vi "Main.vi"() -> ()   [LabVIEW 2020]
doc: "Use this template to build a simple state machine design pattern. Each state executes code and determines which state to transition to."
uses:
  controls/ICM-LOG State.ctl
  controls/ICM-LOG Data.ctl
panel:
  out "Top Label":string
  in  "Tab Control":T1(tab)
  in  "Export definition":bool
  in  "delete definition":bool
  in  "Import definition":bool
  in  "Definition Type":u16(ring) items=["Choose a Definition", "device", "module", "channel", "metric", "instance", "unit", "asset", "datasource", "capability", "camera"]
  in  "Definition List":i32(listbox)
  in  "Export Asset":bool
  in  "Import Asset":bool
  in  "Asset Configuration File Path":path
  in  "Asset":string="Equipment"
  in  "Start Date/Time":timestamp=timestamp(3664461539.734 s since 1904-01-01)
  in  "End Date/Time":timestamp=timestamp(3664465840.411149 s since 1904-01-01)
  in  "Destination Folder":path=path "C:/TDMS_Logs"
  in  "File List":i32(listbox)=-1
  in  "Pull Data":bool
  in  "Exit":bool
  out "Status":string="Exported 0 files to C:\\TDMS_Logs."
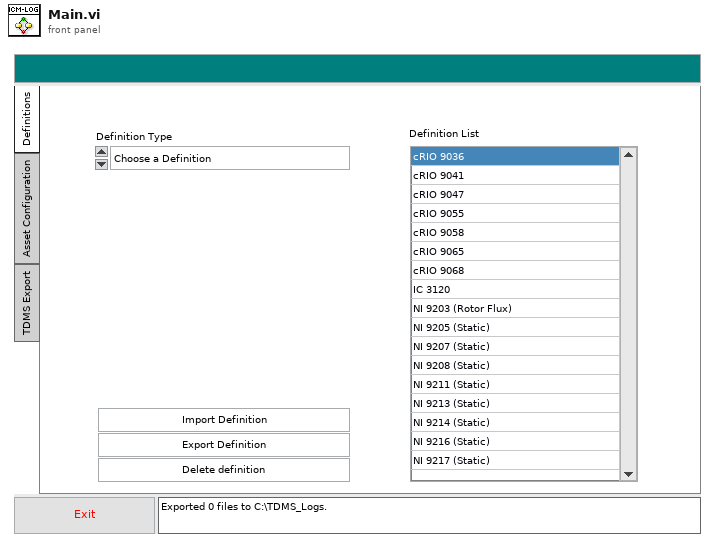
[diagram p1: front panel]
types:
  T1 = enum32{"Definitions", "Asset Configuration", "TDMS Export"}
  T2 = typedef "ICM-LOG Data.ctl" = cluster{"Asset":string, "Start Date/Time":timestamp, "End Date/Time":timestamp, "Destination Folder":path, "Command":string, "Standard Output":string, "filename":string, "Item Name":string, "GUID":string}
  T3 = typedef "ICM-LOG State.ctl" = enum16{"Initialize", "Wait for Event", "List Definitions", "Import Definition", "Export Definition", "Delete Definition", "Export Asset Configuration", "Import Asset Configuration", "Build Command", "Run Command", "Update Definition List", "Update File List", "Open File", "Exit"}
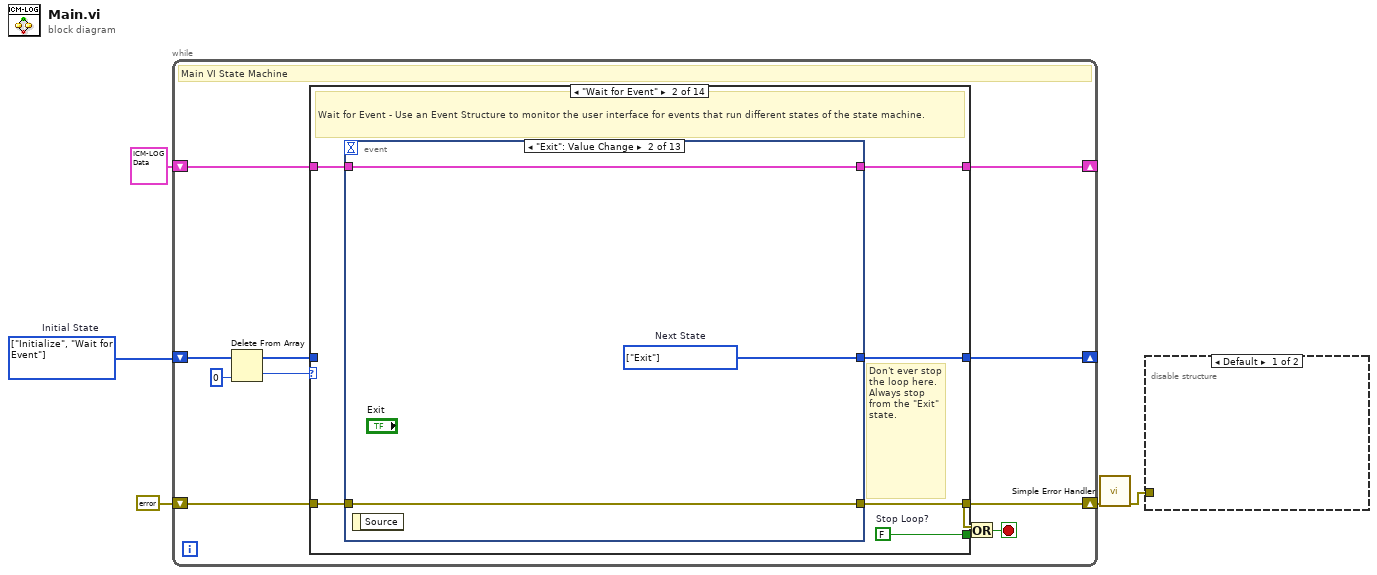
[diagram p0: block diagram]
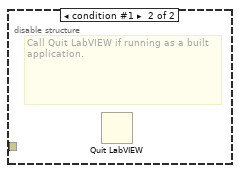
[diagram p2: hidden frame]
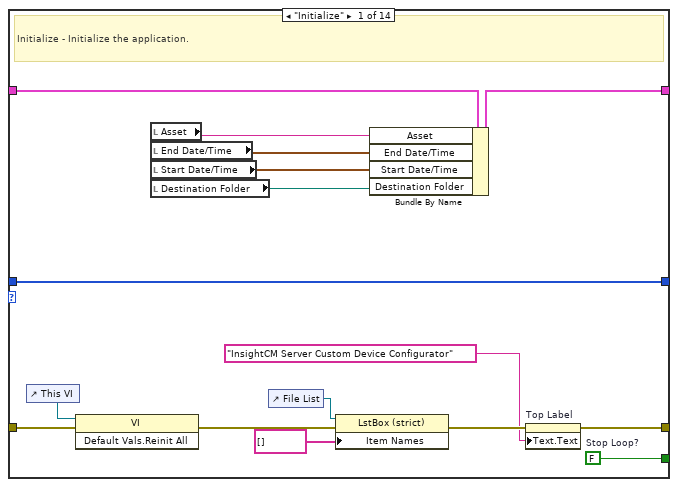
[diagram p3: hidden frame]
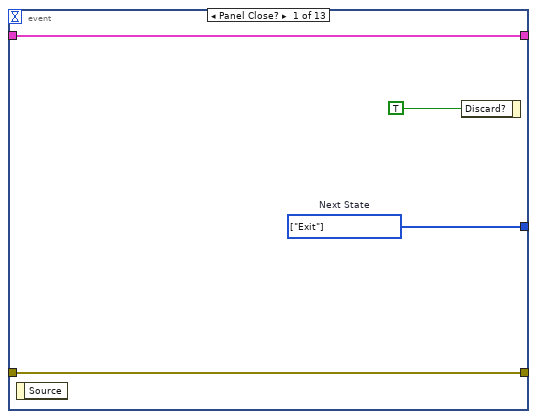
[diagram p4: hidden frame]
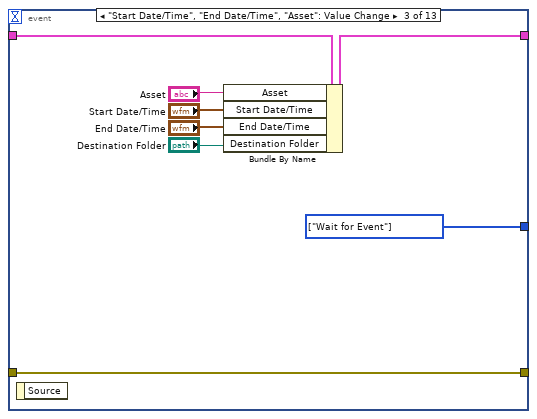
[diagram p5: hidden frame]
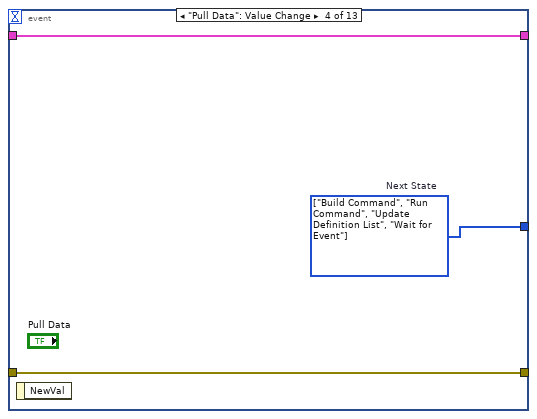
[diagram p6: hidden frame]
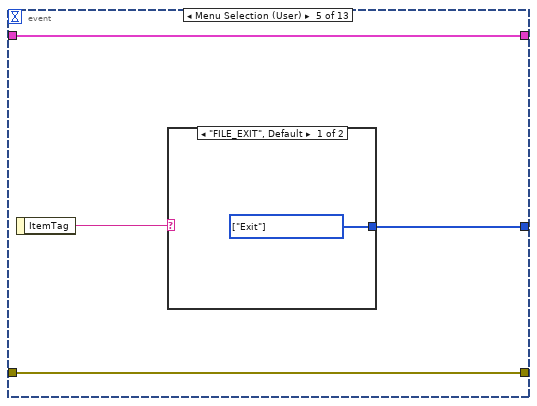
[diagram p7: hidden frame]
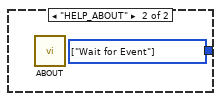
[diagram p8: hidden frame]
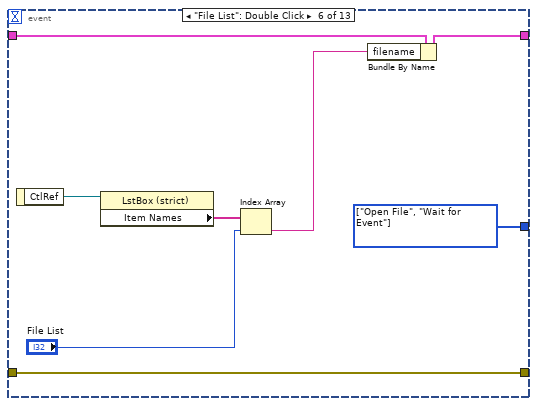
[diagram p9: hidden frame]
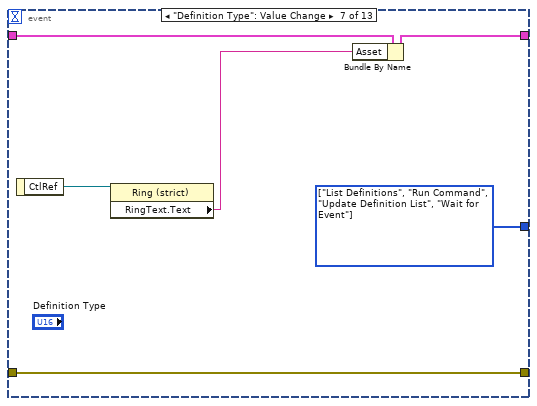
[diagram p10: hidden frame]
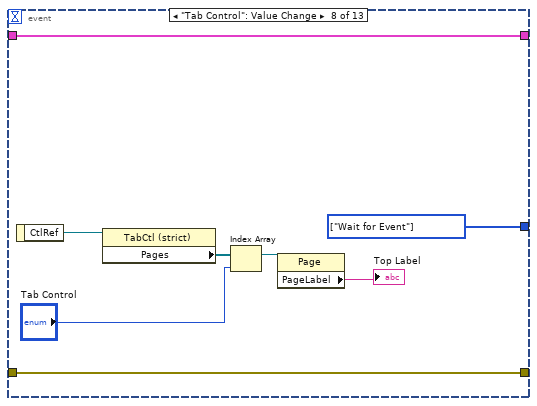
[diagram p11: hidden frame]
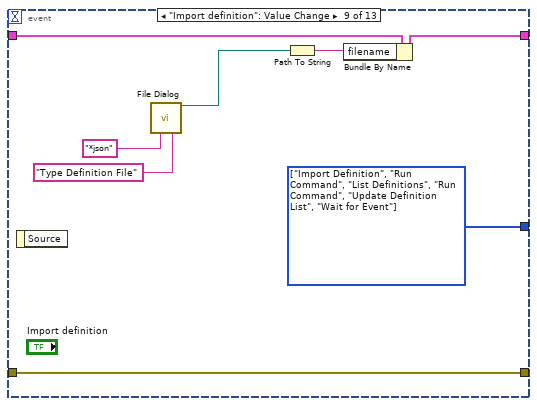
[diagram p12: hidden frame]
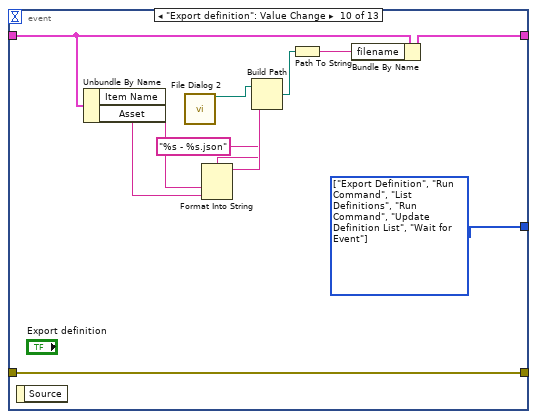
[diagram p13: hidden frame]
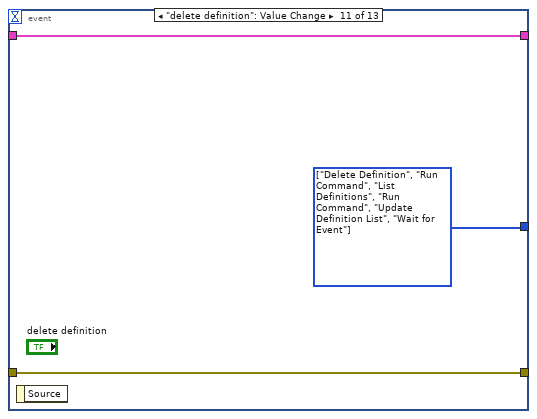
[diagram p14: hidden frame]
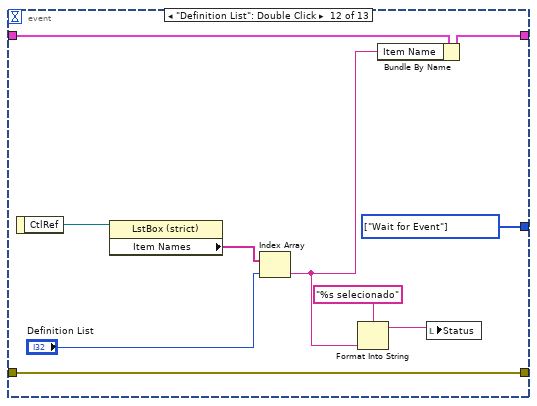
[diagram p15: hidden frame]
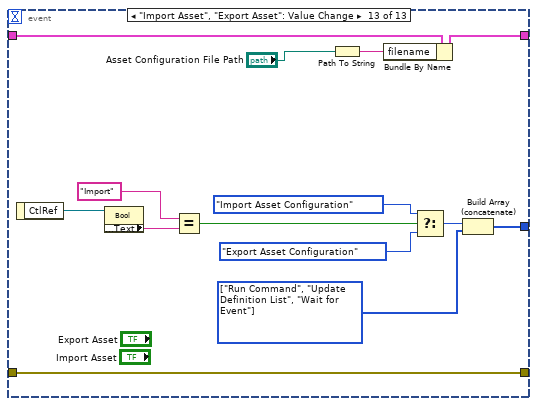
[diagram p16: hidden frame]
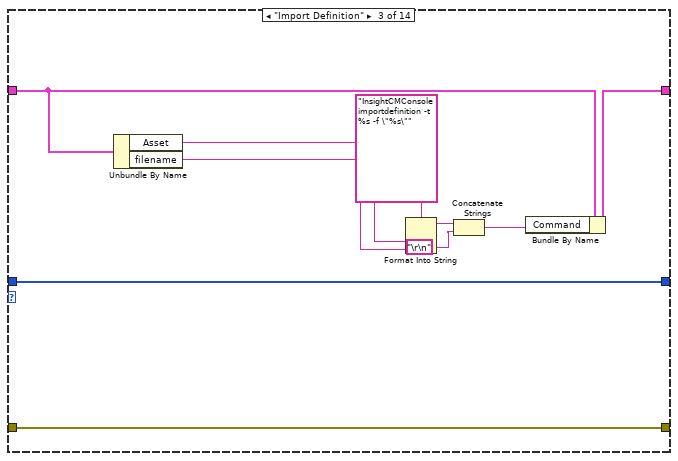
[diagram p17: hidden frame]
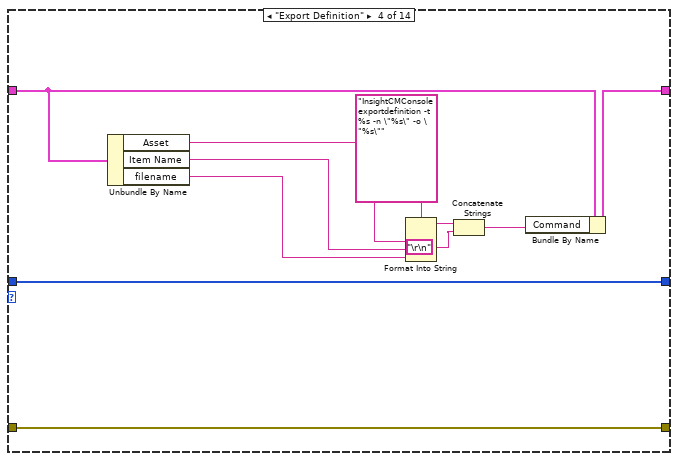
[diagram p18: hidden frame]
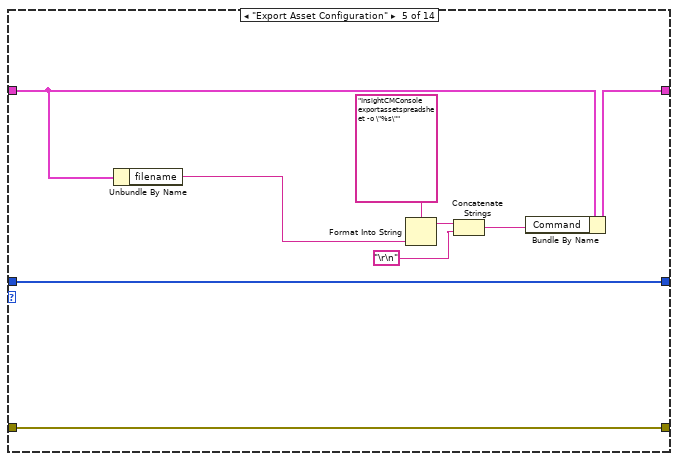
[diagram p19: hidden frame]
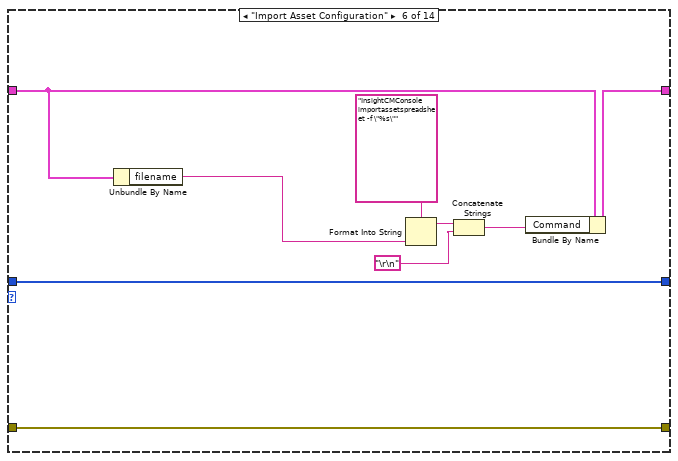
[diagram p20: hidden frame]
diagram:
  w5 = T3[] [enum."Initialize", enum."Wait for Event"] items=["Initialize", "Wait for Event", "List Definitions", "Import Definition", "Export Definition", "Delete Definition", "Export Asset Configuration", "Import Asset Configuration", "Build Command", "Run Command", "Update Definition List", "Update File List", "Open File", "Exit"]  # Initial State
  n1 = while {
    shift-right: [w7] -> _
    shift-left: w5 -> [w10]
    shift-right: [w15] -> _
    shift-left: T2 {"Asset"="", "Start Date/Time"=timestamp(0 s since 1904-01-01), "End Date/Time"=timestamp(0 s since 1904-01-01), "Destination Folder"=path "C:/TDMS_Logs", "Command"="", "Standard Output"="", "filename"="", "Item Name"="", "GUID"=""} ("Data") -> [w16]
    shift-right: [w11] -> w2
    shift-left: errorcluster {"status"=FALSE, "code"=0, "source"=""} ("error constant") -> [w14]
    stop <- w12 stop-if-true
    # "Main VI State Machine"
    n2 = Delete From Array(array=w10, index=0) -> (deleted portion=w9:T3, array with subset deleted=w8:T3[])  [unwired: 1 in]
    n3 = case shown="\"Wait for Event\"" w9 {
      tunnel: [w17 w38 w131 w141 w152 w161 w170 w180 w189 w206 w218 w240 w248 w258] -> w7
      tunnel: [w20 w37 _ _ _ _ _ _ _ FALSE ("Stop Loop?") _ _ _ w256] -> w13
      tunnel: w16 -> [w32 w36 w139 w150 w159 w168 w178 w187 w204 w216 w233 w246 w253 w257]
      tunnel: [w30 w35 w135 w147 w157 w166 w175 w185 w193 w209 w233 w246 w253 w257] -> w15
      tunnel: w14 -> [w31 w34 w140 w151 w160 w169 w179 w188 w205 w213 w234 w247 w254 w255]
      tunnel: [w19 w33 w140 w151 w160 w169 w179 w188 w205 w212 w234 w247 w250 w255] -> w11
      tunnel: w8 -> [w17 _ w131 w141 w152 w161 w170 w180 w189 w206 w218 w240 w248 _]
      frame "Initialize" {
        w20 = FALSE  # Stop Loop?
        # "Initialize - Initialize the application."
        n4 = control-ref of="This VI"() -> (w24:refnum<vi>)
        n5 = invoke class="VI" method="Default Vals.Reinit All"(reference=w24, error in=w31) -> (error out=w25:errorcluster)  [unwired: 1 in, 2 out]
        n6 = local read "Asset"() -> (w29:string)
        n7 = local read "End Date/Time"() -> (w28:timestamp)
        n8 = local read "Start Date/Time"() -> (w27:timestamp)
        n9 = local read "Destination Folder"() -> (w26:path)
        n10 = control-ref of="File List"() -> (w22:refnum<vi>)
        n11 = property class="LstBox (strict)"(reference=w22, error in=w25, "Item Names"=string[] []) -> (error out=w23:errorcluster)  [unwired: 1 out]
        n12 = Bundle By Name(cluster=w32, "Asset"=w29, "End Date/Time"=w28, "Start Date/Time"=w27, "Destination Folder"=w26) -> (w30:T2)
        n13 = property on="Top Label" class="Str"(error in=w23, "Text.Text"="InsightCM Server Custom Device Configurator" ("Top Label")) -> (error out=w19:errorcluster)  [unwired: 1 in, 1 out]
      }
      frame "Wait for Event" {
        w37 = FALSE  # Stop Loop?
        # "Don't ever stop the loop here. Always stop from the \"Exit\" state."
        # "Wait for Event - Use an Event Structure to monitor the user interface for events that run different states of the state machine."
        n14 = event shown="[1] \"Exit\": Value Change" {
          selector: _ -> [_ _ _ _ _ _ _ _ _ _ _ _ _]
          dyn-events: _ -> [_ _ _ _ _ _ _ _ _ _ _ _ _]
          timeout: _ -> [_ _ _ _ _ _ _ _ _ _ _ _ _]
          tunnel: [w42 w45 w46 w56 w57 w68 w74 w77 w89 w93 w104 w107 w117] -> w38
          tunnel: w36 -> [w41 w44 w53 w55 w60 w70 w76 w84 w88 w94 w106 w116 w130]
          tunnel: [w41 w44 w51 w55 w60 w64 w72 w84 w91 w102 w106 w111 w128] -> w35
          tunnel: w34 -> [w40 w43 w52 w54 w59 w69 w75 w83 w92 w103 w105 w115 w129]
          tunnel: [w40 w43 w52 w54 w59 w69 w75 w83 w92 w103 w105 w115 w129] -> w33
          event Panel Close? {
            w42 = T3[] [enum."Exit"] items=["Initialize", "Wait for Event", "List Definitions", "Import Definition", "Export Definition", "Delete Definition", "Export Asset Configuration", "Import Asset Configuration", "Build Command", "Run Command", "Update Definition List", "Update File List", "Open File", "Exit"]  # Next State
            n15 = event-data() -> ()  [unwired: 1 in, 1 out]
            n16 = event-data("Discard?"=TRUE) -> ()  [unwired: 1 in, 1 out]
          }
          event "Exit": Value Change {
            w45 = T3[] [enum."Exit"] items=["Initialize", "Wait for Event", "List Definitions", "Import Definition", "Export Definition", "Delete Definition", "Export Asset Configuration", "Import Asset Configuration", "Build Command", "Run Command", "Update Definition List", "Update File List", "Open File", "Exit"]  # Next State
            n17 = event-data() -> ()  [unwired: 1 in, 1 out]
          }
          event "Start Date/Time", "End Date/Time", "Asset": Value Change {
            w46 = T3[] [enum."Wait for Event"] items=["Initialize", "Wait for Event", "List Definitions", "Import Definition", "Export Definition", "Delete Definition", "Export Asset Configuration", "Import Asset Configuration", "Build Command", "Run Command", "Update Definition List", "Update File List", "Open File", "Exit"] ("Next State")
            n18 = event-data() -> ()  [unwired: 1 in, 1 out]
            n19 = Bundle By Name(cluster=w53, "Asset"="Asset", "Start Date/Time"="Start Date/Time", "End Date/Time"="End Date/Time", "Destination Folder"="Destination Folder") -> (w51:T2)
          }
          event "Pull Data": Value Change {
            w56 = T3[] [enum."Build Command", enum."Run Command", enum."Update Definition List", enum."Wait for Event"] items=["Initialize", "Wait for Event", "List Definitions", "Import Definition", "Export Definition", "Delete Definition", "Export Asset Configuration", "Import Asset Configuration", "Build Command", "Run Command", "Update Definition List", "Update File List", "Open File", "Exit"]  # Next State
            n20 = event-data() -> ()  [unwired: 1 in, 1 out]
          }
          event Menu Selection (User) {
            n21 = event-data() -> ("ItemTag"=w58:string)  [unwired: 1 in]
            n22 = case shown="\"FILE_EXIT\", Default" w58 {
              tunnel: [w61 w62] -> w57
              frame "FILE_EXIT", Default {
                w61 = T3[] [enum."Exit"] items=["Initialize", "Wait for Event", "List Definitions", "Import Definition", "Export Definition", "Delete Definition", "Export Asset Configuration", "Import Asset Configuration", "Build Command", "Run Command", "Update Definition List", "Update File List", "Open File", "Exit"] ("Next State")
              }
              frame "HELP_ABOUT" {
                w62 = T3[] [enum."Wait for Event"] items=["Initialize", "Wait for Event", "List Definitions", "Import Definition", "Export Definition", "Delete Definition", "Export Asset Configuration", "Import Asset Configuration", "Build Command", "Run Command", "Update Definition List", "Update File List", "Open File", "Exit"] ("Next State")
                n23 = call "ABOUT.vi"() -> ()  [unwired: 12 in]
              }
            }
          }
          event "File List": Double Click {
            w68 = T3[] [enum."Open File", enum."Wait for Event"] items=["Initialize", "Wait for Event", "List Definitions", "Import Definition", "Export Definition", "Delete Definition", "Export Asset Configuration", "Import Asset Configuration", "Build Command", "Run Command", "Update Definition List", "Update File List", "Open File", "Exit"] ("Next State")
            n24 = event-data() -> ("CtlRef"=w67:refnum<vi>)  [unwired: 1 in]
            n25 = property class="LstBox (strict)"(reference=w67) -> ("Item Names"=w66:string[])  [unwired: 1 in, 2 out]
            n26 = Index Array(array=w66, index="File List") -> (element=w63:string)
            n27 = Bundle By Name(cluster=w70, "filename"=w63) -> (w64:T2)
          }
          event "Definition Type": Value Change {
            w74 = T3[] [enum."List Definitions", enum."Run Command", enum."Update Definition List", enum."Wait for Event"] items=["Initialize", "Wait for Event", "List Definitions", "Import Definition", "Export Definition", "Delete Definition", "Export Asset Configuration", "Import Asset Configuration", "Build Command", "Run Command", "Update Definition List", "Update File List", "Open File", "Exit"] ("Next State")
            n28 = event-data() -> ("CtlRef"=w73:refnum<vi>)  [unwired: 1 in]
            n29 = property class="Ring (strict)"(reference=w73) -> ("RingText.Text"=w71:string)  [unwired: 1 in, 2 out]
            n30 = Bundle By Name(cluster=w76, "Asset"=w71) -> (w72:T2)
          }
          event "Tab Control": Value Change {
            w77 = T3[] [enum."Wait for Event"] items=["Initialize", "Wait for Event", "List Definitions", "Import Definition", "Export Definition", "Delete Definition", "Export Asset Configuration", "Import Asset Configuration", "Build Command", "Run Command", "Update Definition List", "Update File List", "Open File", "Exit"] ("Next State")
            n31 = event-data() -> ("CtlRef"=w82:refnum<vi>)  [unwired: 1 in]
            n32 = property class="TabCtl (strict)"(reference=w82) -> ("Pages"=w81:refnum<vi>[])  [unwired: 1 in, 2 out]
            n33 = Index Array(array=w81, index="Tab Control") -> (element=w80:refnum<vi>)
            n34 = property class="Page"(reference=w80) -> ("PageLabel"=→"Top Label":string)  [unwired: 1 in, 2 out]
          }
          event "Import definition": Value Change {
            w89 = T3[] [enum."Import Definition", enum."Run Command", enum."List Definitions", enum."Run Command", enum."Update Definition List", enum."Wait for Event"] items=["Initialize", "Wait for Event", "List Definitions", "Import Definition", "Export Definition", "Delete Definition", "Export Asset Configuration", "Import Asset Configuration", "Build Command", "Run Command", "Update Definition List", "Update File List", "Open File", "Exit"] ("Next State")
            n35 = event-data() -> ()  [unwired: 1 in, 1 out]
            n36 = call "File Dialog"("pattern (all files)"="*json", "pattern label"="Type Definition File") -> ("selected path"=w87:path)  [unwired: 10 in, 3 out]
            n37 = Path To String(path=w87) -> (string=w90:string)
            n38 = Bundle By Name(cluster=w88, "filename"=w90) -> (w91:T2)
          }
          event "Export definition": Value Change {
            w93 = T3[] [enum."Export Definition", enum."Run Command", enum."List Definitions", enum."Run Command", enum."Update Definition List", enum."Wait for Event"] items=["Initialize", "Wait for Event", "List Definitions", "Import Definition", "Export Definition", "Delete Definition", "Export Asset Configuration", "Import Asset Configuration", "Build Command", "Run Command", "Update Definition List", "Update File List", "Open File", "Exit"] ("Next State")
            n39 = event-data() -> ()  [unwired: 1 in, 1 out]
            n40 = Unbundle By Name(w94) -> ("Item Name"=w100:string, "Asset"=w99:string)
            n41 = call "File Dialog 2"() -> ("selected path"=w98:path)  [unwired: 12 in, 3 out]
            n42 = Format Into String(format string="%s - %s.json", w100, w99) -> (resulting string=w97:string)  [unwired: 2 in, 1 out]
            n43 = Build Path(base path=w98, name or relative path=w97) -> (appended path=w95:path)
            n44 = Path To String(path=w95) -> (string=w101:string)
            n45 = Bundle By Name(cluster=w94, "filename"=w101) -> (w102:T2)
          }
          event "delete definition": Value Change {
            w104 = T3[] [enum."Delete Definition", enum."Run Command", enum."List Definitions", enum."Run Command", enum."Update Definition List", enum."Wait for Event"] items=["Initialize", "Wait for Event", "List Definitions", "Import Definition", "Export Definition", "Delete Definition", "Export Asset Configuration", "Import Asset Configuration", "Build Command", "Run Command", "Update Definition List", "Update File List", "Open File", "Exit"] ("Next State")
            n46 = event-data() -> ()  [unwired: 1 in, 1 out]
          }
          event "Definition List": Double Click {
            w107 = T3[] [enum."Wait for Event"] items=["Initialize", "Wait for Event", "List Definitions", "Import Definition", "Export Definition", "Delete Definition", "Export Asset Configuration", "Import Asset Configuration", "Build Command", "Run Command", "Update Definition List", "Update File List", "Open File", "Exit"] ("Next State")
            n47 = event-data() -> ("CtlRef"=w114:refnum<vi>)  [unwired: 1 in]
            n48 = property class="LstBox (strict)"(reference=w114) -> ("Item Names"=w113:string[])  [unwired: 1 in, 2 out]
            n49 = Index Array(array=w113, index="Definition List") -> (element=w108:string)
            n50 = Format Into String(format string="%s selecionado", w108) -> (resulting string=w110:string)  [unwired: 2 in, 1 out]
            n51 = Bundle By Name(cluster=w116, "Item Name"=w108) -> (w111:T2)
            n52 = local write "Status"(w110) -> ()
          }
          event "Import Asset", "Export Asset": Value Change {
            w118 = T3[] [enum."Run Command", enum."Update Definition List", enum."Wait for Event"] items=["Initialize", "Wait for Event", "List Definitions", "Import Definition", "Export Definition", "Delete Definition", "Export Asset Configuration", "Import Asset Configuration", "Build Command", "Run Command", "Update Definition List", "Update File List", "Open File", "Exit"] ("Next State")
            n53 = event-data() -> ("CtlRef"=w125:refnum<vi>)  [unwired: 1 in]
            n54 = property class="Bool"(reference=w125) -> ("BoolText.Text"=w122:string)  [unwired: 1 in, 2 out]
            n55 = Equal?(x="Import", y=w122) -> (x = y?=w121:bool)
            n56 = Path To String(path="Asset Configuration File Path") -> (string=w126:string)
            n57 = Bundle By Name(cluster=w130, "filename"=w126) -> (w128:T2)
            n58 = Select(t=ICM-LOG_State."Import Asset Configuration" ("Next State"), s=w121, f=ICM-LOG_State."Export Asset Configuration" ("Next State")) -> (s? t:f=w119:T3)
            n59 = Build Array (concatenate)(w119, w118) -> (w117:T3[])
          }
        }
      }
      frame "Import Definition" {
        n60 = Unbundle By Name(w139) -> ("Asset"=w137:string, "filename"=w136:string)
        n61 = Format Into String(format string="InsightCMConsole importdefinition -t %s -f \"%s\"", w137, w136) -> (resulting string=w134:string)  [unwired: 2 in, 1 out]
        n62 = Concatenate Strings(w134, "\r\n") -> (w133:string)
        n63 = Bundle By Name(cluster=w139, "Command"=w133) -> (w135:T2)
      }
      frame "Export Definition" {
        n64 = Unbundle By Name(w150) -> ("Asset"=w148:string, "Item Name"=w142:string, "filename"=w143:string)
        n65 = Format Into String(format string="InsightCMConsole exportdefinition -t %s -n \"%s\" -o \"%s\"", w148, w142, w143) -> (resulting string=w146:string)  [unwired: 2 in, 1 out]
        n66 = Concatenate Strings(w146, "\r\n") -> (w145:string)
        n67 = Bundle By Name(cluster=w150, "Command"=w145) -> (w147:T2)
      }
      frame "Export Asset Configuration" {
        n68 = Unbundle By Name(w159) -> ("filename"=w153:string)
        n69 = Format Into String(format string="InsightCMConsole exportassetspreadsheet -o \"%s\"", w153) -> (resulting string=w156:string)  [unwired: 2 in, 1 out]
        n70 = Concatenate Strings(w156, "\r\n") -> (w155:string)
        n71 = Bundle By Name(cluster=w159, "Command"=w155) -> (w157:T2)
      }
      frame "Import Asset Configuration" {
        n72 = Unbundle By Name(w168) -> ("filename"=w162:string)
        n73 = Format Into String(format string="InsightCMConsole importassetspreadsheet -f \"%s\"", w162) -> (resulting string=w165:string)  [unwired: 2 in, 1 out]
        n74 = Concatenate Strings(w165, "\r\n") -> (w164:string)
        n75 = Bundle By Name(cluster=w168, "Command"=w164) -> (w166:T2)
      }
      frame "Delete Definition" {
        n76 = Unbundle By Name(w178) -> ("Asset"=w176:string, "Item Name"=w171:string)
        n77 = Format Into String(format string="InsightCMConsole deletedefinition -t %s -n \"%s\"", w176, w171) -> (resulting string=w174:string)  [unwired: 2 in, 1 out]
        n78 = Concatenate Strings(w174, "\r\n") -> (w173:string)
        n79 = Bundle By Name(cluster=w178, "Command"=w173) -> (w175:T2)
      }
      frame "List Definitions" {
        n80 = Unbundle By Name(w187) -> ("Asset"=w181:string)
        n81 = Format Into String(format string="InsightCMConsole listdefinitions -t %s", w181) -> (resulting string=w184:string)  [unwired: 2 in, 1 out]
        n82 = Concatenate Strings(w184, "\r\n") -> (w183:string)
        n83 = Bundle By Name(cluster=w187, "Command"=w183) -> (w185:T2)
      }
      frame "Build Command" {
        n84 = Unbundle By Name(w204) -> ("Destination Folder"=w200:path, "Asset"=w198:string, "Start Date/Time"=w197:timestamp, "End Date/Time"=w196:timestamp)
        n85 = Path To String(path=w200) -> (string=w199:string)
        n86 = Format Date/Time String(time format string (%c)="\"%Y-%m-%d %H:%M:%S\"", seconds (now)=w197) -> (date/time string=w195:string)  [unwired: 1 in]
        n87 = Format Date/Time String(time format string (%c)="\"%Y-%m-%d %H:%M:%S\"", seconds (now)=w196) -> (date/time string=w194:string)  [unwired: 1 in]
        n88 = Format Into String(format string="InsightCMConsole exporttdms -dir %s -asset \"%s\" -start %s -end %s", w199, w198, w195, w194) -> (resulting string=w192:string)  [unwired: 2 in, 1 out]
        n89 = Concatenate Strings(w192, "\r\n") -> (w191:string)
        n90 = Bundle By Name(cluster=w204, "Command"=w191) -> (w193:T2)
      }
      frame "Run Command" {
        w211 = path "C:/Program Files/National Instruments/InsightCM Server 3.0"  # Working Directory
        # "User State 1 - Replace this state with functionality for your own application."
        n91 = Unbundle By Name(w216) -> ("Command"=w210:string)
        n92 = call <vilib>:"System Exec.vi"("run minimized? (F)"=TRUE, "wait until completion? (T)"=TRUE, "error in (no error)"=w213, "working directory"=w211, "standard input"=w210, "command line"="cmd") -> ("error out"=w212:errorcluster, "standard output"=w208:string)  [unwired: 2 in, 2 out]
        n93 = Bundle By Name(cluster=w216, "Standard Output"=w208) -> (w209:T2)
      }
      frame "Update Definition List" {
        # "device, module, channel, metric, instance, unit, asset, datasource, capability, camera"
        n94 = Unbundle By Name(w233) -> ("Standard Output"=w230:string)
        n95 = Spreadsheet String To Array(format string="%s", spreadsheet string=w230, array type (2D Dbl)="") -> (array=w229:string[][])  [unwired: 1 in]
        n96 = Index Array(array=w229, index (col)=0 ("disabled index (col)")) -> (element=w227:string[])  [unwired: 1 in]
        n97 = Delete From Array(array=w227, length=6, index=0) -> (deleted portion=w223:string[], array with subset deleted=w222:string[])
        n98 = Delete From Array(array=w222, length=3) -> (array with subset deleted=w219:string[])  [unwired: 1 in, 1 out]
        n99 = Index Array(array=w223, index=4) -> (element=→"Status":string)
        n100 = property on="Definition List" class="LstBox (strict)"("Item Names"=w219) -> ()  [unwired: 2 in, 2 out]
      }
      frame "Update File List" {
        n101 = Unbundle By Name(w246) -> ("Standard Output"=w243:string, "Destination Folder"=w236:path)
        n102 = Spreadsheet String To Array(format string="%s", spreadsheet string=w243, array type (2D Dbl)="") -> (array=w242:string[][])  [unwired: 1 in]
        n103 = List Folder(path=w236, pattern="*.tdms") -> (filenames=w235:string[])  [unwired: 2 in, 3 out]
        n104 = Index Array(array=w242, index (row)=5 ("disabled index (row)"), index (col)=0 ("disabled index (col)")) -> (element=w238:string)
        n105 = local write "Status"(w238) -> ()
        n106 = property on="File List" class="LstBox (strict)"("Item Names"=w235) -> ()  [unwired: 2 in, 2 out]
      }
      frame "Open File" {
        n107 = Unbundle By Name(w253) -> ("Destination Folder"=w252:path, "filename"=w251:string)
        n108 = Build Path(base path=w252, name or relative path=w251) -> (appended path=w249:path)
        n109 = call <vilib>:"TDMS - File Viewer.vi"("error in (no error)"=w254, "file path"=w249) -> ("error out"=w250:errorcluster)  [unwired: 4 in, 1 out]
      }
      frame "Exit" {
        w256 = TRUE  # Stop Loop?
        w258 = T3[] [enum."Exit"] items=["Initialize", "Wait for Event", "List Definitions", "Import Definition", "Export Definition", "Delete Definition", "Export Asset Configuration", "Import Asset Configuration", "Build Command", "Run Command", "Update Definition List", "Update File List", "Open File", "Exit"]  # (Value Not Used)
        # "#CodeNeeded - Add any required cleanup code here."
        # "The state value is not used here since this is the last iteration of the state machine loop."
        # "Exit - Exit the application."
      }
    }
    n110 = Or(x=w11, y=w13) -> (x .or. y?=w12:bool)
  }
  n111 = call <vilib>:"Simple Error Handler.vi"("error in (no error)"=w2) -> ("error out"=w1:errorcluster)  [unwired: 4 in, 4 out]
  n112 = disable-structure shown="Default" {
    disable-tunnel: w1 -> [_ _]
    frame condition #0 (active) {
    }
    frame condition #1 {
      # "Call Quit LabVIEW if running as a built application."
      n113 = Quit LabVIEW() -> ()  [unwired: 1 in]
    }
  }
